vi "Request Data.vi"(8 "error in":errorcluster, 10 "Message ID":u8) -> (0 "error out":errorcluster, 3 "Response Queue":refnum<queue>)   [LabVIEW 2019, in "Binary Actor.lvlib"]
uses:
  Binary Actor.lvlib
  Actor Command.ctl
  Actor Task.ctl
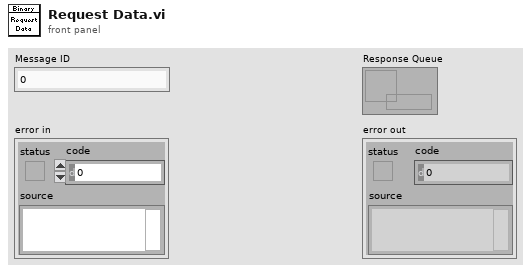
[diagram p1: front panel]
types:
  T1 = typedef "Binary Actor.lvlib/Actor Task.ctl" = enum8{"Write", "Get Data", "Stop"}
  T2 = typedef "Binary Actor.lvlib/Actor Command.ctl" = cluster{"Task":T1, "Data":string, "Response Queue":refnum<queue>}
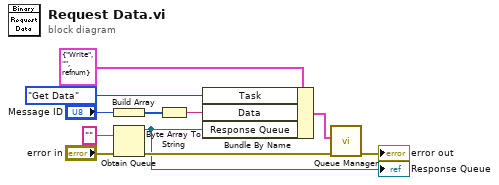
[diagram p0: block diagram]
diagram:
  n1 = Build Array("Message ID") -> (w1:u8[])
  n2 = Obtain Queue(element data type="", error in (no error)="error in") -> (queue out=w4:refnum<queue>, error out=w9:errorcluster)  [unwired: 3 in, 1 out]
  "Response Queue" <- w4
  n3 = Byte Array To String(unsigned byte array=w1) -> (string=w2:string)
  n4 = Bundle By Name(cluster=T2 {"Task"=enum."Write", "Data"="", "Response Queue"=refnum} ("Command"), "Task"=Actor_Task."Get Data", "Data"=w2, "Response Queue"=w4) -> (w6:T2)
  n5 = call "Queue Manager.vi"("error in"=w9, "Command"=w6) -> ("error out"=→"error out":errorcluster)  [unwired: 8 in, 1 out]
